vi "DataSocket Server Control.vi"(4 "error in (no error)":errorcluster, 7 "operation (launch)":enum16{"launch", "show", "hide", "close"}(ring)) -> (0 "error out":errorcluster)   [LabVIEW 2009]
doc: "Performs one of the following operations on the DataSocket server on the local machine:\n\n<B>launch</B> - starts the DataSocket Server.\n<B>show</B> - opens the DataSocket Server window.\n<B>hide</B> - closes the DataSocket Server window.\n<B>close</B> - stops the DataSocket Server."
panel:
  in  "CWDataServer.ICWDataServer":refnum<k7>
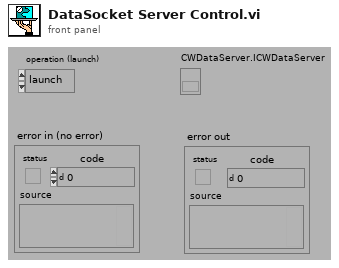
[diagram p1: front panel]
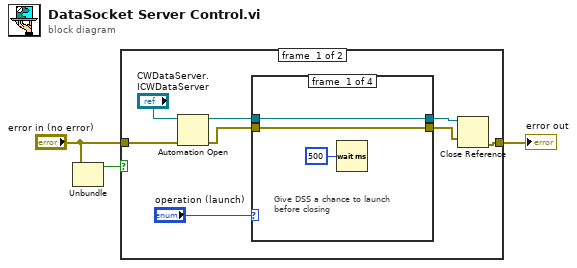
[diagram p0: block diagram]
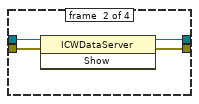
[diagram p2: hidden frame]
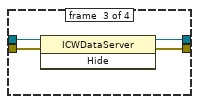
[diagram p3: hidden frame]
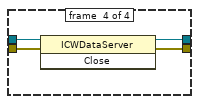
[diagram p4: hidden frame]
diagram:
  n1 = Unbundle("error in (no error)") -> ("status"=w1:bool)  [unwired: 2 out]
  n2 = case shown="False" w1 {
    tunnel: "error in (no error)" -> [w6 w27]
    tunnel: [w4 w27] -> w3
    frame #0 {
      n3 = Automation Open(error in (no error)=w6, Automation Refnum="CWDataServer.ICWDataServer") -> (Automation Refnum=w11:refnum<k7>, error out=w9:errorcluster)  [unwired: 2 in]
      n4 = case shown="\"launch\"" "operation (launch)" {
        tunnel: w11 -> [w12 w18 w22 w26]
        tunnel: [w12 w17 w21 w25] -> w10
        tunnel: w9 -> [w14 w16 w20 w24]
        tunnel: [w14 w15 w19 w23] -> w8
        frame #0 {
          # "Give DSS a chance to launch\nbefore closing"
          n5 = Wait (ms)(milliseconds to wait=u32 500) -> ()  [unwired: 1 out]
        }
        frame #1 {
          n6 = invoke class="ICWDataServer" method="Show"(reference=w18, error in=w16) -> (reference out=w17:refnum<k7>, error out=w15:errorcluster)  [unwired: 1 in, 1 out]
        }
        frame #2 {
          n7 = invoke class="ICWDataServer" method="Hide"(reference=w22, error in=w20) -> (reference out=w21:refnum<k7>, error out=w19:errorcluster)  [unwired: 1 in, 1 out]
        }
        frame #3 {
          n8 = invoke class="ICWDataServer" method="Close"(reference=w26, error in=w24) -> (reference out=w25:refnum<k7>, error out=w23:errorcluster)  [unwired: 1 in, 1 out]
        }
      }
      n9 = Close Reference(reference=w10, error in (no error)=w8) -> (error out=w4:errorcluster)
    }
    frame #1 {
    }
  }
  "error out" <- w3
